vi "_DoubleClickDialog.vi"(8 "error in (no error)":errorcluster, 10 "XRef":T1, 11 "State In":T2) -> (0 "error out":errorcluster, 3 "State Out":T2)   [LabVIEW 2014, in "TagDB(dev).lvlib" / "tagDB_setValue.xnode"]
uses:
  tagDB_setValue.xnode
  State.ctl
  <vilib>/XNodeSupport/XNodeXNodeRef.ctl
  <vilib>/XNodeSupport/NI_XNodeSupport.lvlib
panel:
  out "Type":variant
  out "Cancelled?":bool
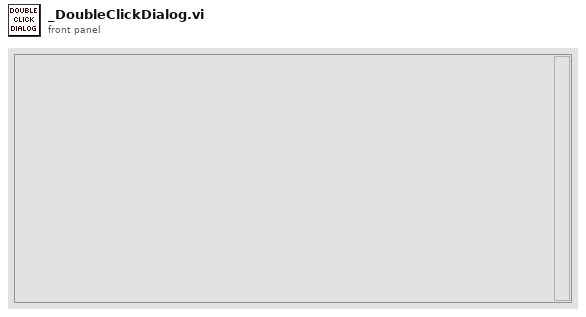
[diagram p1: front panel]
types:
  T1 = typedef "NI_XNodeSupport.lvlib/XNodeXNodeRef.ctl" = refnum<vi>
  T2 = typedef "TagDB(dev).lvlib/tagDB_setValue.xnode/State.ctl" = cluster{"Type":variant}
  T3 = typedef "eventvkey.ctl" = enum16{"ASCII", "Enter", "Return", "Shift", "Ctrl", "Alt", "Cmd", "Opt", "Caps", "NumLock", "Clear", "Break", "Up", "Down", "Left", "Right", "Insert", "Delete", "Home", "End", "PageUp", "PageDown", "Escape", "Help", "Pause", "ScrollLock", "F1", "F2", "F3", "F4", "F5", "F6", "F7", "F8", "F9", "F10", "F11", "F12", "F13", "F14", "F15", "F16", "F17", "F18", "F19", "F20", "F21", "F22", "F23", "F24", "Play", "VolumeUp", "VolumeDown", "Mute", "Two Byte Char"}
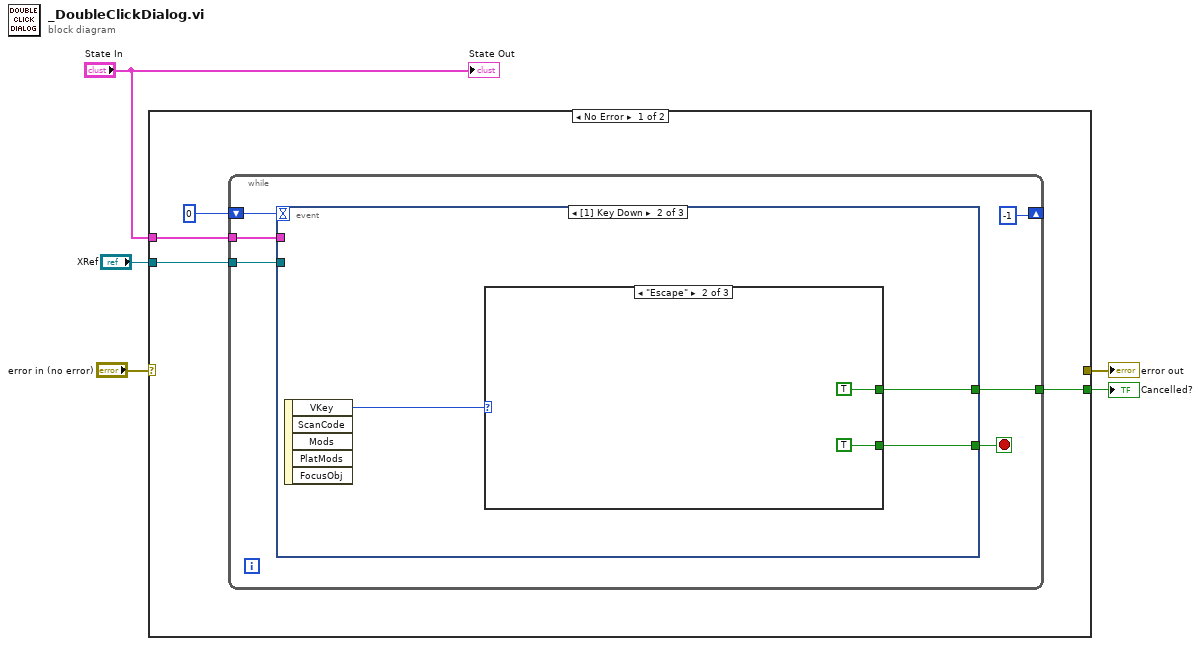
[diagram p0: block diagram]
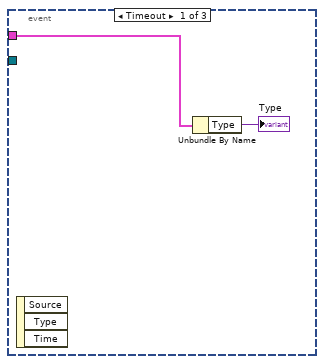
[diagram p2: hidden frame]
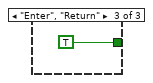
[diagram p4: hidden frame]
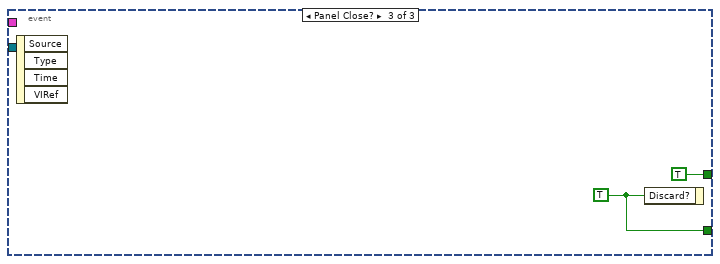
[diagram p5: hidden frame]
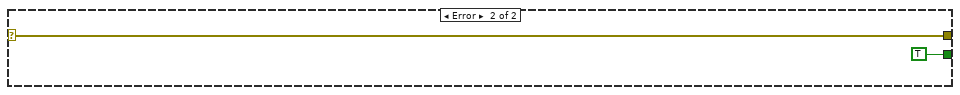
[diagram p6: hidden frame]
diagram:
  n1 = case shown="No Error" "error in (no error)" {
    selector: "error in (no error)" -> [_ w27]
    tunnel: [w8 TRUE] -> w5
    tunnel: [_ w27] -> w3
    tunnel: "State In" -> [w7 _]
    tunnel: "XRef" -> [w6 _]
    frame No Error {
      n2 = while {
        shift-right: [-1] -> _
        shift-left: 0 -> [w14]
        tunnel: [w12] -> w8
        tunnel: w7 -> [w11]
        tunnel: w6 -> [w10]
        stop <- w15 stop-if-true
        n3 = event shown="[1] Key Down" {
          selector: _ -> [_ _ _]
          dyn-events: _ -> [_ _ _]
          timeout: w14 -> [_ _ _]
          tunnel: [_ w19 w25] -> w15
          tunnel: [_ w18 TRUE] -> w12
          tunnel: w11 -> [w17 _ _]
          tunnel: w10 -> [_ _ _]
          event Timeout {
            n4 = event-data() -> ()  [unwired: 1 in, 3 out]
            n5 = Unbundle By Name(w17) -> ("Type"=→"Type":variant)
          }
          event Key Down {
            n6 = event-data() -> ("VKey"=w20:T3)  [unwired: 1 in, 4 out]
            n7 = case shown="\"Escape\"" w20 {
              tunnel: [_ TRUE TRUE] -> w19
              tunnel: [_ TRUE _] -> w18
              frame Default {
              }
              frame "Escape" {
              }
              frame "Enter", "Return" {
              }
            }
          }
          event Panel Close? {
            w25 = TRUE ("Discard?")
            n8 = event-data() -> ()  [unwired: 1 in, 4 out]
            n9 = event-data("Discard?"=w25) -> ()  [unwired: 1 in, 1 out]
          }
        }
      }
    }
    frame Error {
    }
  }
  "Cancelled?" <- w5
  "error out" <- w3
  "State Out" <- "State In"
